vi "QueryTxUp.vi"(3 "error in (no error)":errorcluster) -> (0 "error out":errorcluster, 1 "String_TxDetVoltage":string, 2 "IfTransmittingOne":i32, 5 "Volts Tx Detector":dbl)   [LabVIEW 2009]
doc: "compare the voltage from the crystal detector to a fixed value of 0.0005 volts, if greater, then the tx is operating."
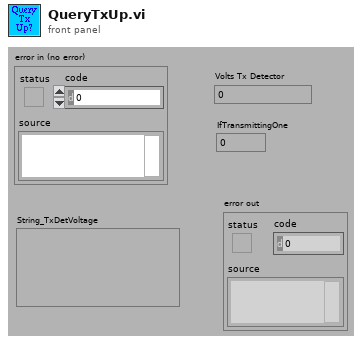
[diagram p1: front panel]
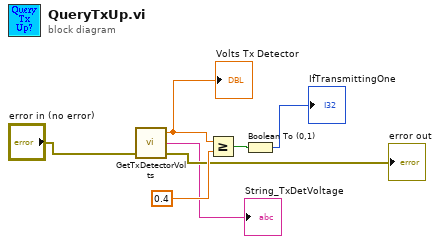
[diagram p0: block diagram]
diagram:
  n1 = call "GetTxDetectorVolts.vi"("error in (no error)"="error in (no error)") -> ("error out"=→"error out":errorcluster, "String_Volts_TxDet"=→"String_TxDetVoltage":string, "Volts Tx Detector"=w2:dbl)  [unwired: 2 in]
  "Volts Tx Detector" <- w2
  n2 = Greater Or Equal?(x=w2, y=0.4) -> (x >= y?=w4:bool)
  n3 = Boolean To (0,1)(Boolean=w4) -> (0, 1=→"IfTransmittingOne":i16)
